vi "Script_Excit_Build_From_Wfms.vi"(8 "error in (no error)":errorcluster, 9 "Number of excitations":i32=1 min=0 max=5 step=1, 10 "Table of Waveforms":string[](array[string]), 11 "Script Path":path=path "D:/PIRENEA/EXCIT_SCRIPTS") -> (0 "error out":errorcluster, 2 "Script File":string="Adiabatic.txt", 3 "Script Text":string)   [LabVIEW 2017]
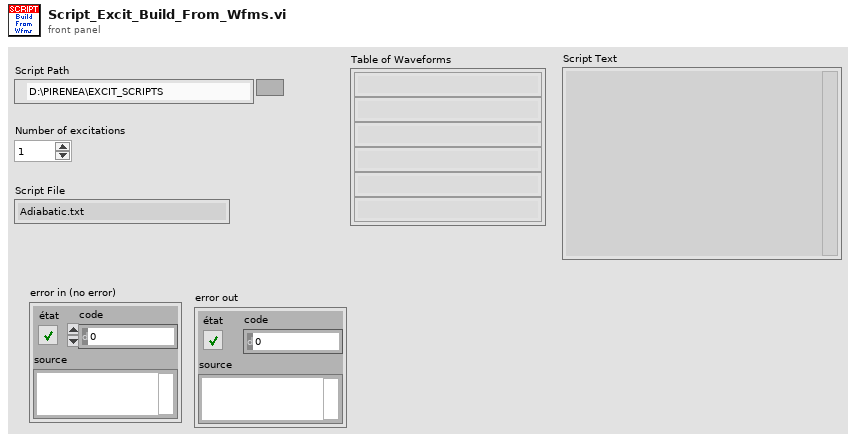
[diagram p1: front panel]
types:
  T1 = enum16{"open", "replace", "create", "open or create", "replace or create", "replace or create with confirmation"}
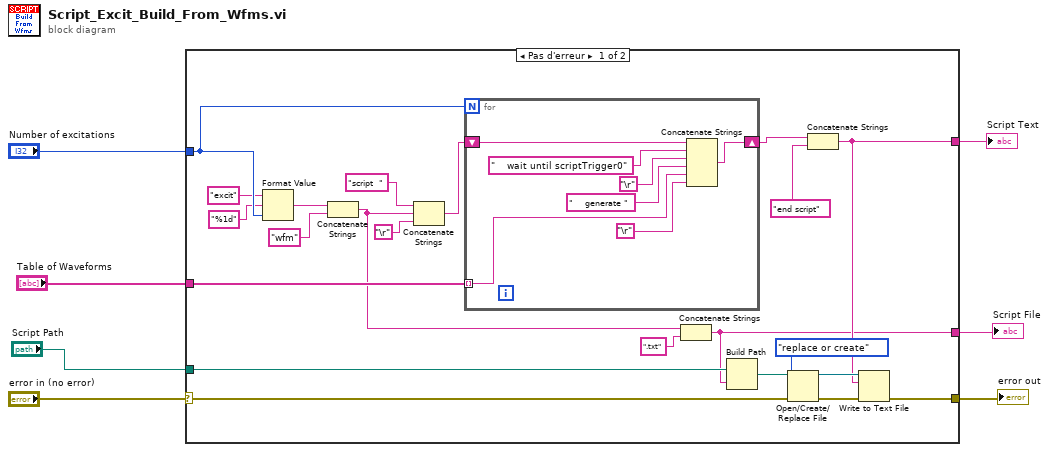
[diagram p0: block diagram]
diagram:
  n1 = case shown="Pas d'erreur" "error in (no error)" {
    selector: "error in (no error)" -> [w16 w37]
    tunnel: [w9 w37] -> w6
    tunnel: "Script Path" -> [w22 _]
    tunnel: "Table of Waveforms" -> [w27 _]
    tunnel: "Number of excitations" -> [w28 _]
    tunnel: [w10 _] -> w2
    tunnel: [w8 _] -> w1
    frame No Error {
      n2 = Format Value(string ("")="excit" ("chaîne"), format string="%1d" ("chaîne de format"), value (0)=w28) -> (output string=w24:string)
      n3 = Concatenate Strings(w24, "wfm" ("chaîne")) -> (w11:string)
      n4 = Concatenate Strings("script  " ("chaîne (\"\")"), w11, "\r") -> (w17:string)
      n5 = for {
        N: w28 -> [_]
        tunnel: w27 -> [w34] mode=indexing
        shift-right: [w32] -> w26
        shift-left: w17 -> [w36]
        n6 = Concatenate Strings(w36, "    wait until scriptTrigger0", "\r", "    generate ", w34, "\r") -> (w32:string)
      }
      n7 = Concatenate Strings(w11, ".txt" ("chaîne")) -> (w8:string)
      n8 = Build Path(base path=w22, name or relative path=w8) -> (appended path=w15:path)
      n9 = Open/Create/Replace File(file path (use dialog)=w15, error in=w16, operation (0:open)=T1."replace or create" ("opération (0 : open)")) -> (refnum out=w13:refnum<file>, error out=w12:errorcluster)  [unwired: 3 in, 1 out]
      n10 = Concatenate Strings(w26, "end script" ("chaîne")) -> (w10:string)
      n11 = Write to Text File(file (use dialog)=w13, text=w10, error in=w12) -> (error out=w9:errorcluster)  [unwired: 1 in, 2 out]
    }
    frame Error {
    }
  }
  "error out" <- w6
  "Script File" <- w1
  "Script Text" <- w2
